vi "parse response string.vi"(8 "error in (no error)":errorcluster, 11 "Rsp str in":string="RPT = 3402\r") -> (0 "error out":errorcluster, 1 "invalid response":bool, 2 "int value":i32=3402, 3 "int string value":string, 5 "String after equal char":string=" 3402")   [LabVIEW 2020]
panel:
  # "response should end with \\r"
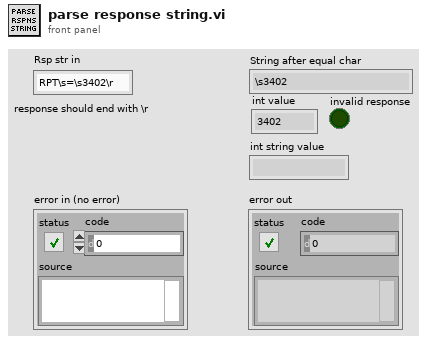
[diagram p1: front panel]
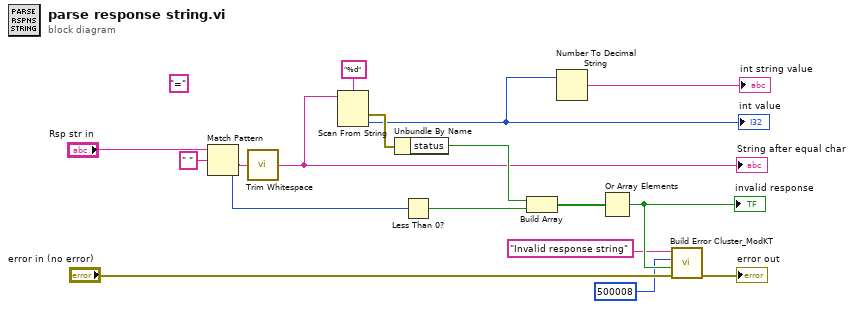
[diagram p0: block diagram]
diagram:
  (unwired) "=" ("regular expression")
  n1 = Match Pattern(string="Rsp str in", regular expression=" ") -> (after substring=w5:string, offset past match=w14:i32)  [unwired: 1 in, 2 out]
  n2 = call <vilib>:"Trim Whitespace.vi"("string"=w5) -> ("trimmed string"=w4:string)  [unwired: 1 in]
  "String after equal char" <- w4
  n3 = Scan From String(format string="%d", input string=w4) -> (error out=w15:errorcluster, output 1=w2:i32)  [unwired: 3 in, 2 out]
  "int value" <- w2
  n4 = Unbundle By Name(w15) -> ("status"=w13:bool)
  n5 = Less Than 0?(x=w14) -> (x < 0?=w12:bool)
  n6 = Build Array(w13, w12) -> (w11:bool[])
  n7 = Number To Decimal String(number=w2) -> (decimal integer string=→"int string value":string)  [unwired: 1 in]
  n8 = Or Array Elements(Boolean array=w11) -> (logical OR=w8:bool)
  "invalid response" <- w8
  n9 = call <vilib>:"Build Error Cluster_ModKT .vi"("Prepend String (\"\")"="Invalid response string" ("Prepend String (\"\")"), "code"=500008, "error? (F)"=w8, "error in (no error)"="error in (no error)") -> ("error out"=→"error out":errorcluster)  [unwired: 3 in, 1 out]
